vi "Vision Processing.vi"(4 "error in (no error)":errorcluster, 7 "Image Size":T1=enum."320x240") -> ()   [LabVIEW 2018]
doc: "This VI runs in parallel to other tasks. It gets images from the camera, processes them for color or shape and use that information to affect robot behavior."
uses:
  <vilib>/Rock Robotics/WPI/Camera/WPI_CameraImageSize.ctl
  <vilib>/Rock Robotics/WPI/Camera/WPI_CameraWhite Balance Values.ctl
  <vilib>/Rock Robotics/WPI/Camera/WPI_CameraExposure Values.ctl
  <vilib>/Rock Robotics/WPI/Camera/WPI_CameraFrameRate.ctl
  Robot Global Data.vi
  <vilib>/vision/NI_Vision_Development_Module.lvlib
panel:
  in  "Lum":cluster{"Lower value":i32, "Upper value":i32}={"Lower value"=30, "Upper value"=100}
  in  "Sat":cluster{"Lower value":i32, "Upper value":i32}={"Lower value"=130, "Upper value"=255}
  in  "Hue":cluster{"Lower value":i32, "Upper value":i32}={"Lower value"=70, "Upper value"=130}
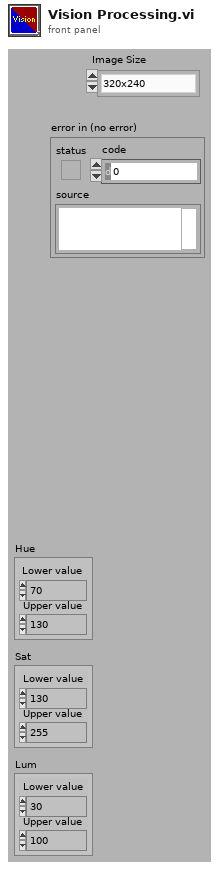
[diagram p1: front panel]
types:
  T1 = typedef "WPI_CameraImageSize.ctl" = enum16{"640x480", "320x240", "160x120", "Custom"}
  T2 = typedef "WPI_CameraFrameRate.ctl" = u32
  T3 = typedef "WPI_CameraExposure Values.ctl" = enum16{"Auto", "Flicker-free 50 Hz", "Flicker-free 60 Hz", "Hold current", "Custom"}
  T4 = typedef "WPI_CameraWhite Balance Values.ctl" = enum16{"Auto", "Fixed indoor", "Fixed outdoor 1", "Fixed outdoor 2", "Fixed fluorescent 1", "Fixed fluorescent 2", "Hold current", "Custom"}
  T5 = typedef "WPI_CameraDevRef.ctl" = cluster{"Camera Address":string, "CameraStatus":errorcluster}
  T6 = typedef "IMAQ Image.ctl" = refnum<image>
  T7 = typedef "Particle Parameters" = i32
  T8 = cluster{"Measurement Parameter":T7, "Range Lower Value":dbl, "Range Upper Value":dbl, "Range":bool, "Measurement Type":bool}[]
  T9 = typedef "Image Type" = u32
  T10 = cluster{"Area":dbl, "Number of Holes":dbl, "Bounding Rect":cluster{"Left":dbl, "Top":dbl, "Right":dbl, "Bottom":dbl}, "Center of Mass":cluster{"X":dbl, "Y":dbl}, "Orientation":dbl, "Dimensions":cluster{"Width":dbl, "Height":dbl}}[]
  T11 = cluster{"Area":dbl, "Number of Holes":dbl, "Bounding Rect":cluster{"Left":dbl, "Top":dbl, "Right":dbl, "Bottom":dbl}, "Center of Mass":cluster{"X":dbl, "Y":dbl}, "Orientation":dbl, "Dimensions":cluster{"Width":dbl, "Height":dbl}}
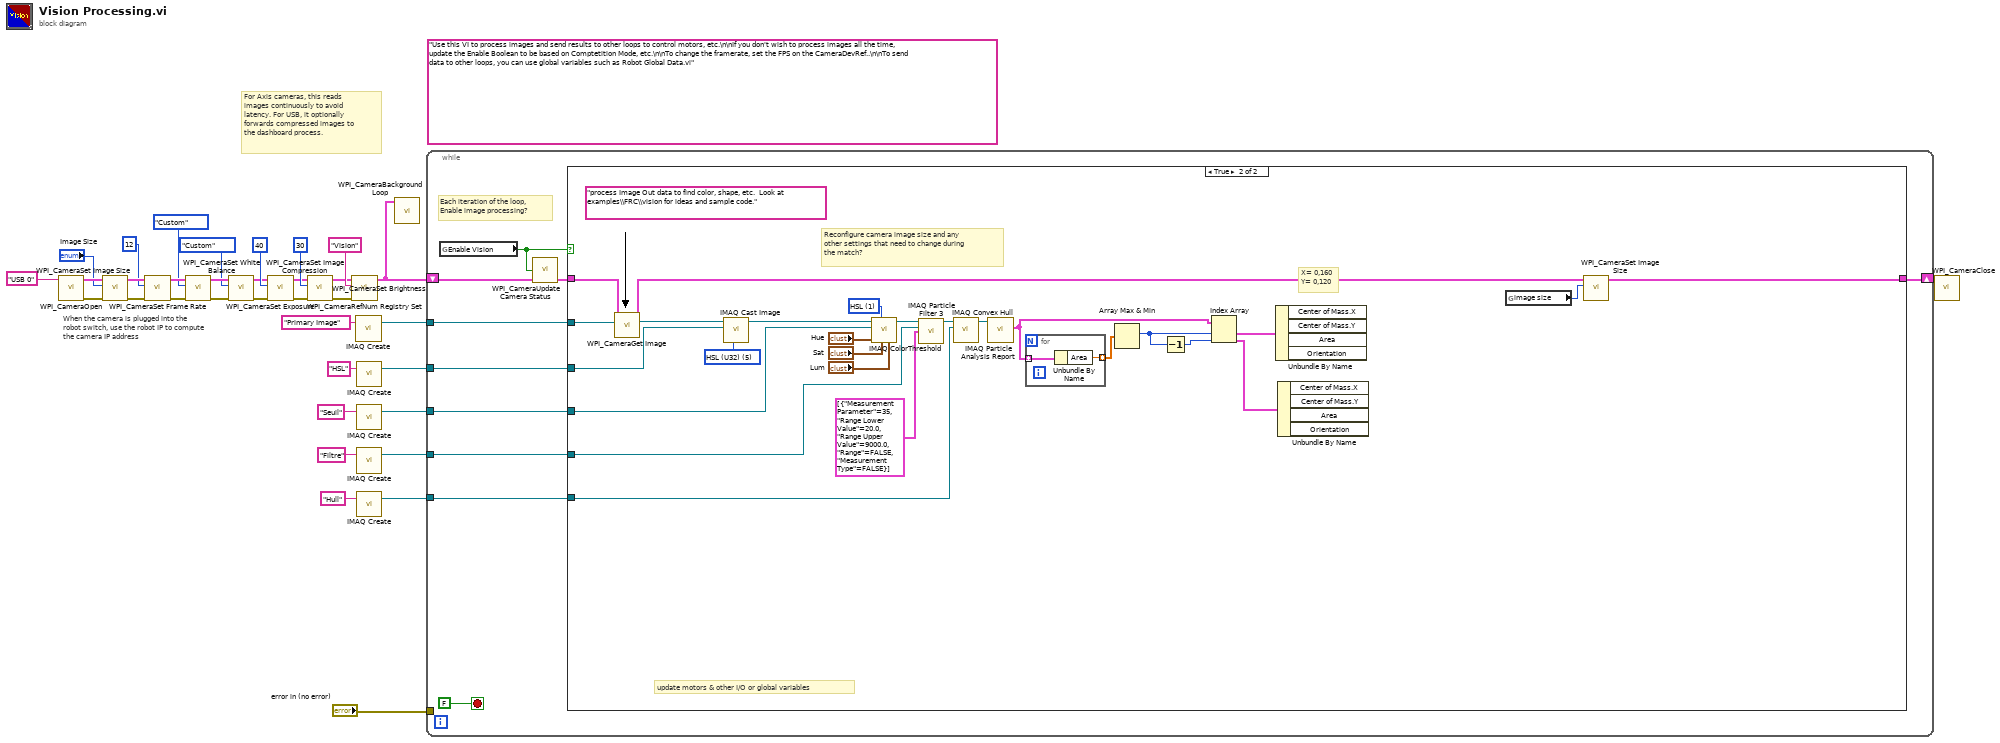
[diagram p0: block diagram]
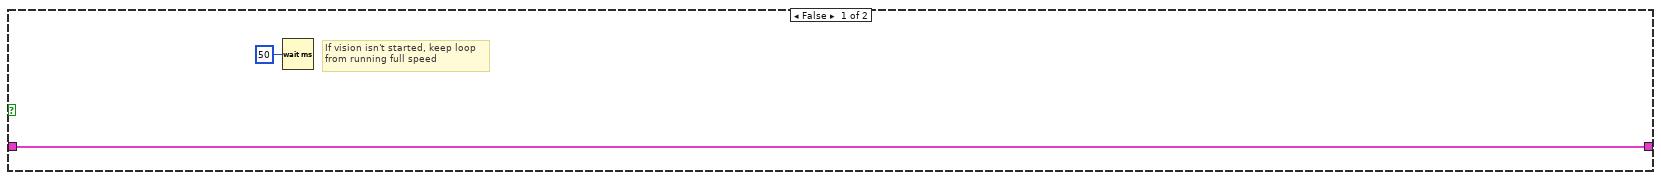
[diagram p2: hidden frame]
diagram:
  (unwired) "Use this VI to process images and send results to other loops to control motors, etc.\n\nIf you don't wish to process images all the time, update the Enable Boolean to be based on Comptetition Mode, etc.\n\nTo change the framerate, set the FPS on the CameraDevRef..\n\nTo send data to other loops, you can use global variables such as Robot Global Data.vi"
  # "When the camera is plugged into the\nrobot switch, use the robot IP to compute\nthe camera IP address"
  # "For Axis cameras, this reads\nimages continuously to avoid\nlatency. For USB, it optionally\nforwards compressed images to\nthe dashboard process."
  n1 = call <vilib>:"WPI_CameraOpen.vi"("Camera Address"="USB 0" ("format string")) -> ("error out"=w24:errorcluster, "CameraDevRef"=w25:T5)  [unwired: 1 in, 8 out]
  n2 = call <vilib>:"WPI_CameraSet Image Size.vi"("error in (no error)"=w24, "Image Size"="Image Size", "CameraDevRef"=w25) -> ("error out"=w23:errorcluster, "CameraDevRef Out"=w26:T5)  [unwired: 1 in, 6 out]
  n3 = call <vilib>:"WPI_CameraSet Frame Rate.vi"("error in (no error)"=w23, "Frame Rate (fps)"=T2 12, "CameraDevRef"=w26) -> ("error out"=w22:errorcluster, "CameraDevRef Out"=w28:T5)  [unwired: 7 out]
  n4 = call <vilib>:"WPI_CameraSet White Balance.vi"("error in (no error)"=w22, "White Balance"=WPI_CameraWhite_Balance_Values."Custom", "CameraDevRef"=w28) -> ("error out"=w21:errorcluster, "CameraDevRef Out"=w27:T5)  [unwired: 1 in, 6 out]
  n5 = call <vilib>:"WPI_CameraSet Exposure.vi"("error in (no error)"=w21, "Exposure"=WPI_CameraExposure_Values."Custom", "CameraDevRef"=w27) -> ("error out"=w20:errorcluster, "CameraDevRef Out"=w30:T5)  [unwired: 1 in, 6 out]
  n6 = call <vilib>:"WPI_CameraSet Image Compression.vi"("error in (no error)"=w20, "Compression"=40, "CameraDevRef"=w30) -> ("error out"=w19:errorcluster, "CameraDevRef Out"=w29:T5)  [unwired: 7 out]
  n7 = call <vilib>:"WPI_CameraSet Brightness.vi"("error in (no error)"=w19, "Brightness"=30, "CameraDevRef"=w29) -> ("error out"=w17:errorcluster, "CameraDevRef Out"=w18:T5)  [unwired: 1 in, 6 out]
  n8 = call <vilib>:"WPI_CameraRefNum Registry Set.vi"("error in (no error)"=w17, "refnum name"="Vision", "CameraDevRef"=w18) -> ("CameraDevRef"=w13:T5)  [unwired: 1 in, 7 out]
  n9 = call "IMAQ Create"("Image Name"="Primary Image") -> ("New Image"=w34:T6)  [unwired: 3 in, 2 out]
  n10 = call "IMAQ Create"("Image Name"="HSL") -> ("New Image"=w4:T6)  [unwired: 3 in, 2 out]
  n11 = call "IMAQ Create"("Image Name"="Seuil") -> ("New Image"=w3:T6)  [unwired: 3 in, 2 out]
  n12 = call "IMAQ Create"("Image Name"="Filtre") -> ("New Image"=w2:T6)  [unwired: 3 in, 2 out]
  n13 = call "IMAQ Create"("Image Name"="Hull") -> ("New Image"=w1:T6)  [unwired: 3 in, 2 out]
  n14 = call <vilib>:"WPI_CameraBackground Loop.vi"("CameraDevRef"=w13) -> ()  [unwired: 11 in]
  n15 = while {
    shift-right: [w44] -> w11
    shift-left: w13 -> [w42]
    tunnel: w34 -> [w43]
    tunnel: "error in (no error)" -> [_]
    tunnel: w4 -> [w39]
    tunnel: w3 -> [w38]
    tunnel: w2 -> [w37]
    tunnel: w1 -> [w36]
    stop <- FALSE stop-if-true
    # "Each iteration of the loop,\nEnable image processing?"
    n16 = global read "Robot Global Data.vi" "Enable Vision"() -> (w40:bool)
    n17 = call <vilib>:"WPI_CameraUpdate Camera Status.vi"("CameraDevRef In"=w42, "Enable Vision"=w40) -> ("CameraDevRef Out"=w41:T5)  [unwired: 3 in]
    n18 = case shown="True" w40 {
      tunnel: w43 -> [_ w72]
      tunnel: [w47 w73] -> w44
      tunnel: w41 -> [w47 w70]
      tunnel: w39 -> [_ w55]
      tunnel: w38 -> [_ w54]
      tunnel: w37 -> [_ w53]
      tunnel: w36 -> [_ w52]
      frame False {
        # "If vision isn't started, keep loop\nfrom running full speed"
        n19 = Wait (ms)(milliseconds to wait=u32 50) -> ()  [unwired: 1 out]
      }
      frame True {
        w60 = u16 1 items=["RGB", "HSL", "HSV", "HSI"] ("Color Mode")
        w59 = T9 5 items=["Grayscale (U8)", "Grayscale (I16)", "Grayscale (SGL)", "Complex (CSG)", "RGB (U32)", "HSL (U32)", "RGB (U64)", "Grayscale (U16)"] ("Image Type")
        (unwired) "process Image Out data to find color, shape, etc.  Look at examples\\FRC\\vision for ideas and sample code."
        # "X= 0,160\nY= 0,120"
        # "update motors & other I/O or global variables"
        # "Reconfigure camera image size and any\nother settings that need to change during\nthe match?"
        n20 = call <vilib>:"WPI_CameraGet Image.vi"("Image"=w72, "CameraDevRef"=w70) -> ("Image Out"=w56:T6, "CameraDevRef Out"=w69:T5)  [unwired: 1 in, 7 out]
        n21 = call "IMAQ Cast Image"("Image Type"=w59, "Image Dst"=w55, "Image Src"=w56) -> ("Image Dst Out"=w61:T6)  [unwired: 7 in, 1 out]
        n22 = call "IMAQ ColorThreshold"("Blue or Luma or Val or Inten Range"="Lum", "Green or Sat Range"="Sat", "Color Mode"=w60, "Red or Hue Range"="Hue", "Image Dst"=w54, "Image Src"=w61) -> ("Image Dst Out"=w65:T6)  [unwired: 4 in, 1 out]
        n23 = call "IMAQ Particle Filter 3"("Image Src"=w65, "Image Dst"=w53, "Selection Values"=T8 [{"Measurement Parameter"=35, "Range Lower Value"=20.0, "Range Upper Value"=9000.0, "Range"=FALSE, "Measurement Type"=FALSE}]) -> ("Image Dst Out"=w62:T6)  [unwired: 10 in, 2 out]
        n24 = call "IMAQ Convex Hull"("Image Dst"=w52, "Image Src"=w62) -> ("Image Dst Out"=w63:T6)  [unwired: 8 in, 1 out]
        n25 = call "IMAQ Particle Analysis Report"("Image"=w63) -> ("Particle Reports (Pixels)"=w57:T10)  [unwired: 5 in, 5 out]
        n26 = for {
          tunnel: w57 -> [w75] mode=indexing
          tunnel: [w74] -> w58 mode=indexing
          n27 = Unbundle By Name(w75) -> ("Area"=w74:dbl)
        }
        n28 = Array Max & Min(array=w58) -> (max index (indices)=w51:i32)  [unwired: 3 out]
        n29 = Decrement(x=w51) -> (x-1=w50:i32)
        n30 = Index Array(array=w57, index #1=w51, index #2=w50) -> (element #1=w49:T11, element #2=w48:T11)
        n31 = Unbundle By Name(w49) -> ()  [unwired: 4 out]
        n32 = Unbundle By Name(w48) -> ()  [unwired: 4 out]
        n33 = global read "Robot Global Data.vi" "image size"() -> (w71:T1)
        n34 = call <vilib>:"WPI_CameraSet Image Size.vi"("Image Size"=w71, "CameraDevRef"=w69) -> ("CameraDevRef Out"=w73:T5)  [unwired: 2 in, 7 out]
      }
    }
  }
  n35 = call <vilib>:"WPI_CameraClose.vi"("CameraDevRef"=w11) -> ()  [unwired: 1 in, 10 out]
